vi "Example Graph.vi"() -> ()   [LabVIEW 2010]
uses:
  C:/tf/play/labview/Tinkerforge.dll
  Tinkerforge.dll
panel:
  in  "stop":bool
  out "graph":cluster{"z":sgl[]}[](graph)
  in  "uid":string="amb"
  in  "port":i32=4223
  in  "host":string="localhost"
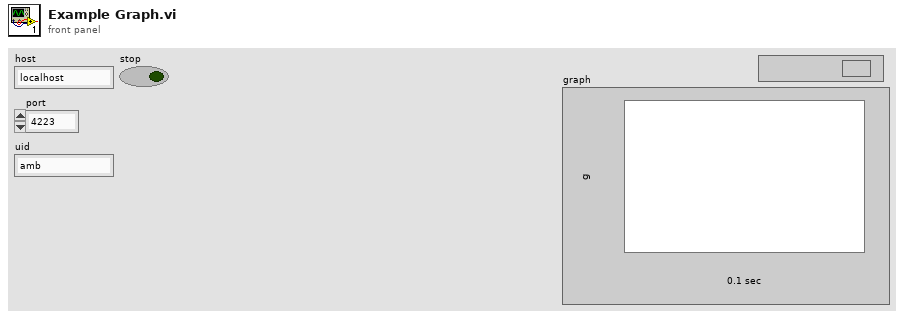
[diagram p1: front panel]
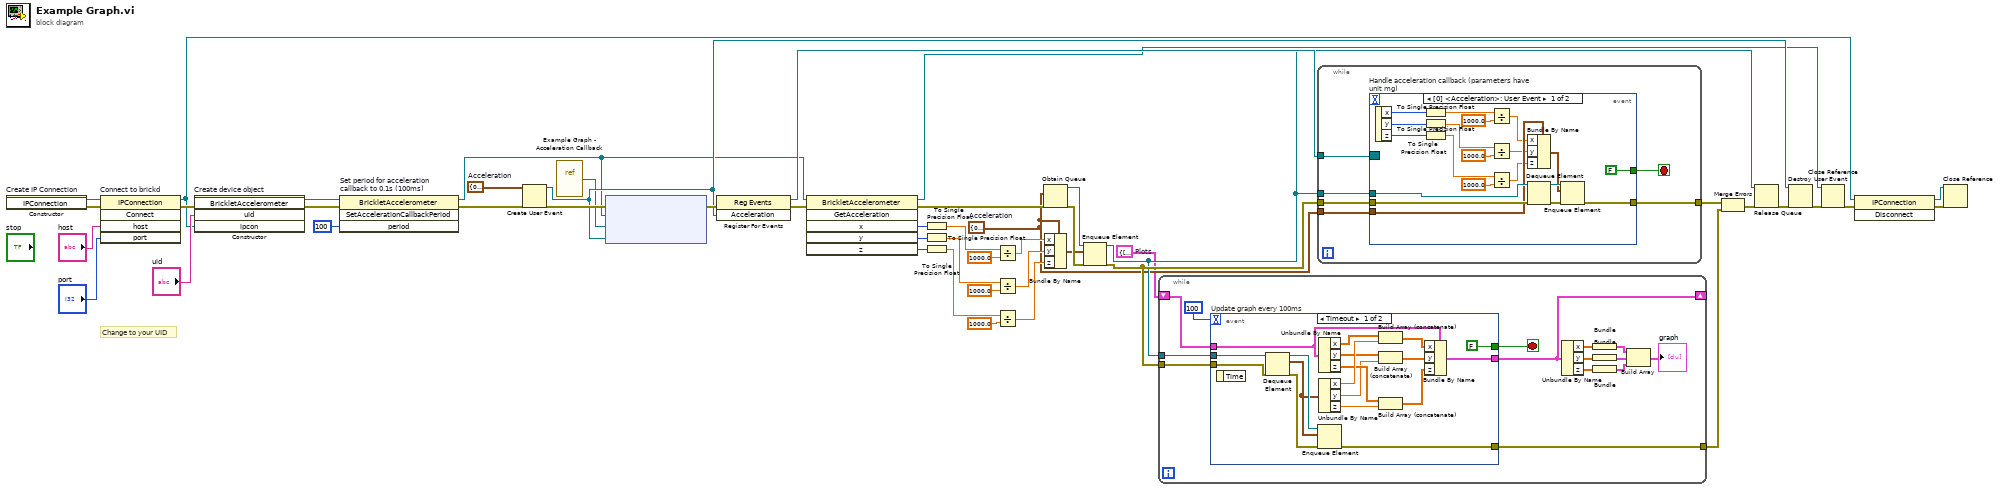
[diagram p0: block diagram]
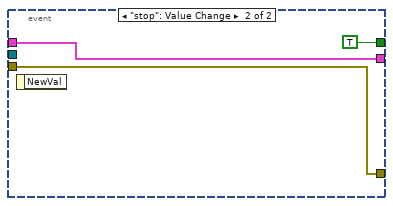
[diagram p2: hidden frame]
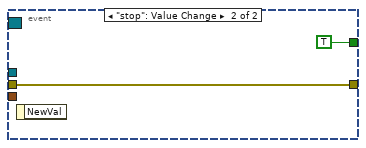
[diagram p3: hidden frame]
diagram:
  w1 = cluster{"x":sgl[], "y":sgl[], "z":sgl[]} {"x"=[], "y"=[], "z"=[]}  # Plots
  w2 = cluster{"x":sgl, "y":sgl, "z":sgl} {"x"=0.0, "y"=0.0, "z"=0.0}  # Acceleration
  w34 = cluster{"x":i16, "y":i16, "z":i16} {"x"=0, "y"=0, "z"=0}  # Acceleration
  # "Change to your UID"
  n1 = constructor on="Create IP Connection" class="IPConnection"() -> (reference out=w48:refnum<k24>, error out=w21:errorcluster)  [unwired: 3 in, 1 out]
  n2 = invoke on="Connect to brickd" class="IPConnection" method="Connect"(reference=w48, error in=w21, "host"="host", "port"="port") -> (reference out=w41:refnum<k24>, error out=w44:errorcluster)  [unwired: 1 in, 3 out]
  n3 = constructor on="Create device object" class="BrickletAccelerometer"(error in=w44, "uid"="uid", "ipcon"=w41) -> (reference out=w31:refnum<k24>, error out=w33:errorcluster)  [unwired: 2 in, 3 out]
  n4 = invoke on="Set period for acceleration\ncallback to 0.1s (100ms)" class="BrickletAccelerometer" method="SetAccelerationCallbackPeriod"(reference=w31, error in=w33, "period"=i64 100) -> (reference out=w18:refnum<k24>, error out=w32:errorcluster)  [unwired: 1 in, 2 out]
  n5 = Create User Event(user event datatype=w34, error in=w32) -> (user event=w36:refnum<user-event>, error out=w39:errorcluster)
  n6 = vi-ref "Example Graph - Acceleration Callback.vi"() -> ("vi reference"=w14:refnum<vi>)
  n7 = node ("Register Event Callback")(w39, w18, w14, w36) -> (w38:errorcluster)  [unwired: 1 in, 1 out]
  n8 = register-events(error in=w38, w36) -> (reference out=w37:refnum<event-registration>, error out=w20:errorcluster)  [unwired: 1 in]
  n9 = invoke class="BrickletAccelerometer" method="GetAcceleration"(reference=w18, error in=w20) -> (reference out=w17:refnum<k24>, error out=w19:errorcluster, "x"=w11:i16, "y"=w4:i16, "z"=w3:i16)  [unwired: 4 in, 1 out]
  n10 = To Single Precision Float(number=w11) -> (single precision float=w16:sgl)
  n11 = To Single Precision Float(number=w4) -> (single precision float=w10:sgl)
  n12 = To Single Precision Float(number=w3) -> (single precision float=w8:sgl)
  n13 = Divide(x=w16, y=sgl 1000.0) -> (x/y=w12:sgl)
  n14 = Divide(x=w10, y=sgl 1000.0) -> (x/y=w5:sgl)
  n15 = Divide(x=w8, y=sgl 1000.0) -> (x/y=w6:sgl)
  n16 = Obtain Queue(element data type=w2, error in (no error)=w19) -> (queue out=w25:refnum<queue>, error out=w27:errorcluster)  [unwired: 3 in, 1 out]
  n17 = Bundle By Name(cluster=w2, "x"=w12, "y"=w5, "z"=w6) -> (w13:cluster{"x":sgl, "y":sgl, "z":sgl})
  n18 = Enqueue Element(queue=w25, element=w13, error in (no error)=w27) -> (queue out=w22:refnum<queue>, error out=w26:errorcluster)  [unwired: 1 in, 1 out]
  n19 = while {
    tunnel: [w59] -> w29
    tunnel: w26 -> [w60]
    shift-right: [w56] -> _
    shift-left: w1 -> [w61]
    tunnel: w22 -> [w58]
    stop <- w57 stop-if-true
    n20 = event "Update graph every 100ms" shown="[0] Timeout" {
      selector: _ -> [_ _]
      dyn-events: _ -> [_ _]
      timeout: 100 -> [_ _]
      tunnel: [w72 w82] -> w56
      tunnel: w61 -> [w73 w82]
      tunnel: w60 -> [w80 w81]
      tunnel: [w77 w81] -> w59
      tunnel: w58 -> [w79 _]
      tunnel: [FALSE TRUE] -> w57
      event Timeout {
        n21 = event-data() -> ()  [unwired: 1 in, 1 out]
        n22 = Dequeue Element(queue=w79, error in (no error)=w80) -> (queue out=w76:refnum<queue>, element=w74:cluster{"x":sgl, "y":sgl, "z":sgl}, error out=w78:errorcluster)  [unwired: 1 in, 1 out]
        n23 = Enqueue Element(queue=w76, element=w74, error in (no error)=w78) -> (error out=w77:errorcluster)  [unwired: 1 in, 2 out]
        n24 = Unbundle By Name(w73) -> ("x"=w71:sgl[], "y"=w68:sgl[], "z"=w65:sgl[])
        n25 = Unbundle By Name(w74) -> ("x"=w70:sgl, "y"=w64:sgl, "z"=w63:sgl)
        n26 = Build Array (concatenate)(w71, w70) -> (w69:sgl[])
        n27 = Build Array (concatenate)(w68, w64) -> (w67:sgl[])
        n28 = Build Array (concatenate)(w65, w63) -> (w66:sgl[])
        n29 = Bundle By Name(cluster=w73, "x"=w69, "y"=w67, "z"=w66) -> (w72:cluster{"x":sgl[], "y":sgl[], "z":sgl[]})
      }
      event "stop": Value Change {
        n30 = event-data() -> ()  [unwired: 1 in, 1 out]
      }
    }
    n31 = Unbundle By Name(w56) -> ("x"=w55:sgl[], "y"=w53:sgl[], "z"=w51:sgl[])
    n32 = Bundle("x"=w55) -> (w54:cluster{"x":sgl[]})  [unwired: 1 in]
    n33 = Bundle("y"=w53) -> (w52:cluster{"y":sgl[]})  [unwired: 1 in]
    n34 = Bundle("z"=w51) -> (w50:cluster{"z":sgl[]})  [unwired: 1 in]
    n35 = Build Array(w54, w52, w50) -> (→"graph":cluster{"z":sgl[]}[])
  }
  n36 = while {
    tunnel: w37 -> [w89]
    tunnel: [w87] -> w28
    tunnel: w26 -> [w88]
    tunnel: w22 -> [w86]
    tunnel: w2 -> [w84]
    stop <- w85 stop-if-true
    n37 = event "Handle acceleration callback (parameters have unit mg)" shown="[0] <Acceleration>: User Event" {
      selector: w89 -> [_ _]
      dyn-events: _ -> [_ _]
      timeout: _ -> [_ _]
      tunnel: w88 -> [w106 w110]
      tunnel: [w104 w110] -> w87
      tunnel: w86 -> [w103 _]
      tunnel: [FALSE TRUE] -> w85
      tunnel: w84 -> [w99 _]
      event User Event {
        n38 = event-data() -> ("x"=w107:i16, "y"=w94:i16, "z"=w91:i16)  [unwired: 1 in]
        n39 = To Single Precision Float(number=w107) -> (single precision float=w108:sgl)
        n40 = To Single Precision Float(number=w94) -> (single precision float=w96:sgl)
        n41 = To Single Precision Float(number=w91) -> (single precision float=w92:sgl)
        n42 = Divide(x=w108, y=sgl 1000.0) -> (x/y=w98:sgl)
        n43 = Divide(x=w96, y=sgl 1000.0) -> (x/y=w95:sgl)
        n44 = Divide(x=w92, y=sgl 1000.0) -> (x/y=w90:sgl)
        n45 = Dequeue Element(queue=w103, error in (no error)=w106) -> (queue out=w102:refnum<queue>, error out=w105:errorcluster)  [unwired: 1 in, 2 out]
        n46 = Bundle By Name(cluster=w99, "x"=w98, "y"=w95, "z"=w90) -> (w100:cluster{"x":sgl, "y":sgl, "z":sgl})
        n47 = Enqueue Element(queue=w102, element=w100, error in (no error)=w105) -> (error out=w104:errorcluster)  [unwired: 1 in, 2 out]
      }
      event "stop": Value Change {
        n48 = event-data() -> ()  [unwired: 1 in, 1 out]
      }
    }
  }
  n49 = Merge Errors(w28, w29) -> (w24:errorcluster)
  n50 = Release Queue(queue=w22, error in (no error)=w24) -> (error out=w23:errorcluster)  [unwired: 1 in, 2 out]
  n51 = Destroy User Event(user event=w36, error in=w23) -> (error out=w35:errorcluster)
  n52 = Close Reference(reference=w17, error in (no error)=w35) -> (error out=w43:errorcluster)
  n53 = invoke class="IPConnection" method="Disconnect"(reference=w41, error in=w43) -> (reference out=w40:refnum<k24>, error out=w42:errorcluster)  [unwired: 1 in, 1 out]
  n54 = Close Reference(reference=w40, error in (no error)=w42) -> ()  [unwired: 1 out]
